vi "StreamReceiveInstrument.vi"() -> ()   [LabVIEW 2018]
panel:
  in  "stop 2":bool
  out "error out":errorcluster
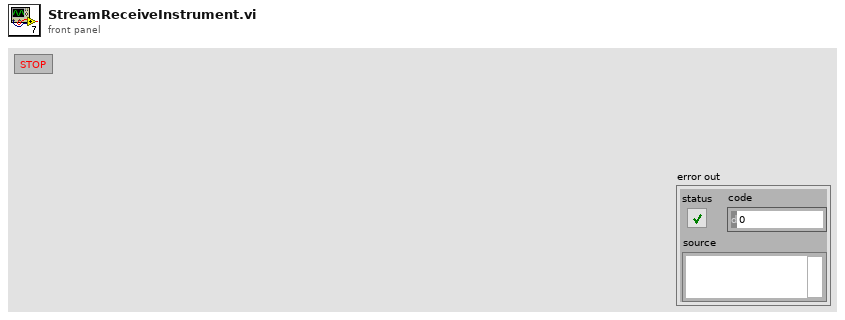
[diagram p1: front panel]
types:
  T1 = cluster{"ID":u32, "Address":string, "Service Name 1":string, "Service Name 2":string, "queue TX":refnum<queue>, "queue RX":refnum<queue>, "Port 1":u32, "Port 2":u32}
  T2 = enum16{"Standard", "Buffered", "CRLF", "Immediate"}
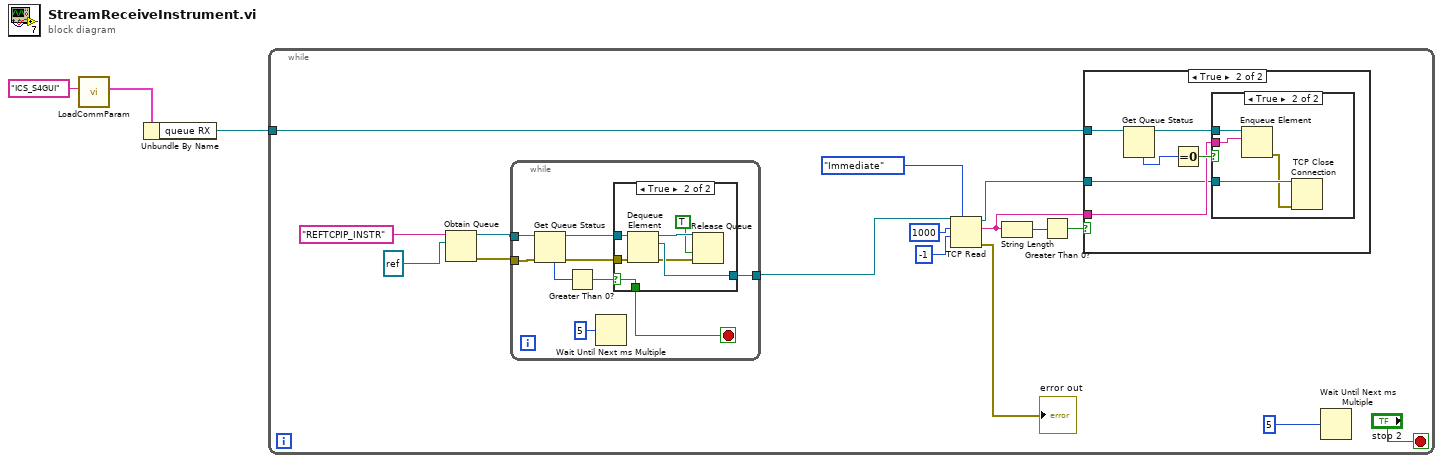
[diagram p0: block diagram]
diagram:
  n1 = call "LoadCommParam.vi"("section name"="ICS_S4GUI") -> ("output cluster"=w3:T1)  [unwired: 10 in]
  n2 = Unbundle By Name(w3) -> ("queue RX"=w1:refnum<queue>)
  n3 = while {
    tunnel: w1 -> [w18]
    stop <- "stop 2" stop-if-true
    n4 = Obtain Queue(name (unnamed)="REFTCPIP_INSTR", element data type=refnum<k5> refnum ("connection ID out")) -> (queue out=w5:refnum<queue>, error out=w4:errorcluster)  [unwired: 3 in, 1 out]
    n5 = while {
      tunnel: [w23] -> w8
      tunnel: w5 -> [w22]
      tunnel: w4 -> [w21]
      stop <- w24 stop-if-true
      n6 = Get Queue Status(queue=w22, error in (no error)=w21) -> (queue out=w28:refnum<queue>, error out=w27:errorcluster, # elements in queue=w25:i32)  [unwired: 1 in, 5 out]
      n7 = Greater Than 0?(x=w25) -> (x > 0?=w26:bool)
      n8 = Wait Until Next ms Multiple(millisecond multiple=u32 5) -> ()  [unwired: 1 out]
      n9 = case shown="True" w26 {
        selector: w26 -> [w29 w34]
        tunnel: w28 -> [_ w36]
        tunnel: w27 -> [_ w35]
        tunnel: [w29 w34] -> w24
        tunnel: [_ w33] -> w23
        frame False {
        }
        frame True {
          n10 = Dequeue Element(queue=w36, error in (no error)=w35) -> (queue out=w32:refnum<queue>, element=w33:refnum<k5>, error out=w31:errorcluster)  [unwired: 1 in, 1 out]
          n11 = Release Queue(queue=w32, force destroy? (F)=TRUE, error in (no error)=w31) -> ()  [unwired: 3 out]
        }
      }
    }
    n12 = TCP Read(connection ID=w8, bytes to read=1000, 7:T2."Immediate" ("mode (standard)"), 9:-1 ("bytes to read")) -> (connection ID out=w9:refnum<k5>, data out=w14:string, error out=→"error out":errorcluster)  [unwired: 1 in]
    n13 = String Length(string=w14) -> (length=w16:i32)
    n14 = Greater Than 0?(x=w16) -> (x > 0?=w15:bool)
    n15 = case shown="True" w15 {
      tunnel: w18 -> [_ w40]
      tunnel: w14 -> [_ w38]
      tunnel: w9 -> [_ w37]
      frame False {
      }
      frame True {
        n16 = Get Queue Status(queue=w40) -> (queue out=w39:refnum<queue>, # elements in queue=w42:i32)  [unwired: 2 in, 6 out]
        n17 = Equal To 0?(x=w42) -> (x = 0?=w41:bool)
        n18 = case shown="True" w41 {
          tunnel: w39 -> [_ w46]
          tunnel: w38 -> [_ w45]
          tunnel: w37 -> [_ w44]
          frame False {
          }
          frame True {
            n19 = Enqueue Element(queue=w46, element=w45) -> (error out=w43:errorcluster)  [unwired: 2 in, 2 out]
            n20 = TCP Close Connection(connection ID=w44, error in (no error)=w43) -> ()  [unwired: 1 in, 2 out]
          }
        }
      }
    }
    n21 = Wait Until Next ms Multiple(millisecond multiple=u32 5) -> ()  [unwired: 1 out]
  }
